vi "Get Node Attribute Value.vi"(8 "error in (no error)":errorcluster, 9 "Attribute Name":string, 11 "Node In":refnum<k20>) -> (0 "error out":errorcluster, 1 "Attribute Refnum":refnum<k20>, 3 "Node Out":refnum<k20>)   [LabVIEW 2014]
uses:
  <vilib>/xml/Close Reference(NNMap).vi
  <resource>/objmgr/DOMUserDefRef.rc
  <vilib>/xml/NI_XML.lvlib
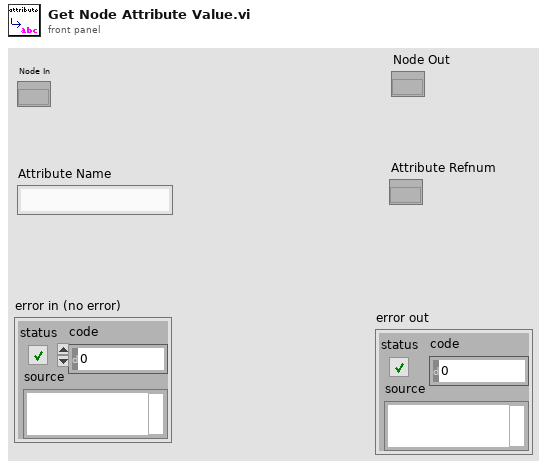
[diagram p1: front panel]
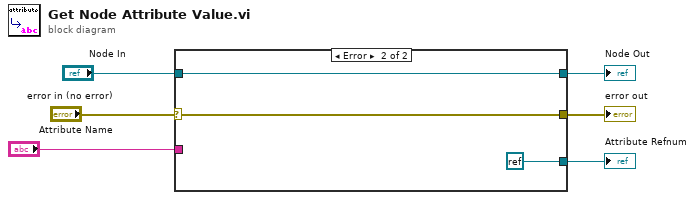
[diagram p0: block diagram]
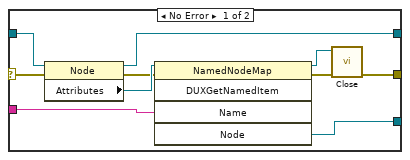
[diagram p2: hidden frame]
diagram:
  n1 = case shown="Error" "error in (no error)" {
    selector: "error in (no error)" -> [w11 w19]
    tunnel: "Node In" -> [w12 w18]
    tunnel: [w9 w18] -> w4
    tunnel: "Attribute Name" -> [w16 _]
    tunnel: [w7 w19] -> w2
    tunnel: [w10 refnum<k0> refnum] -> w1
    frame No Error {
      n2 = property class="Node"(reference=w12, error in=w11) -> (reference out=w9:refnum<k20>, error out=w14:errorcluster, "Attributes"=w15:refnum<k20>)
      n3 = invoke class="NamedNodeMap" method="DUXGetNamedItem"(reference=w15, error in=w14, "Name"=w16) -> (reference out=w13:refnum<k20>, error out=w8:errorcluster, "Node"=w10:refnum<k20>)  [unwired: 2 in, 2 out]
      n4 = call-poly <vilib>:"Close.vi"("error in (no error)"=w8, "named node map"=w13) -> ("error out"=w7:errorcluster)  [unwired: 7 in]
    }
    frame Error {
    }
  }
  "Node Out" <- w4
  "error out" <- w2
  "Attribute Refnum" <- w1
